vi "Set Voltage.vi"(8 "error in (no error)":errorcluster, 10 "Voltage":dbl, 11 "BenchParent in":refnum<class "BenchParent.lvclass">) -> (0 "error out":errorcluster, 3 "BenchParent out":refnum<class "BenchParent.lvclass">)   [LabVIEW 2024, in "BenchParent.lvclass"]
uses:
  BenchParent.lvclass
  BenchParent.lvclass/BenchParent.ctl
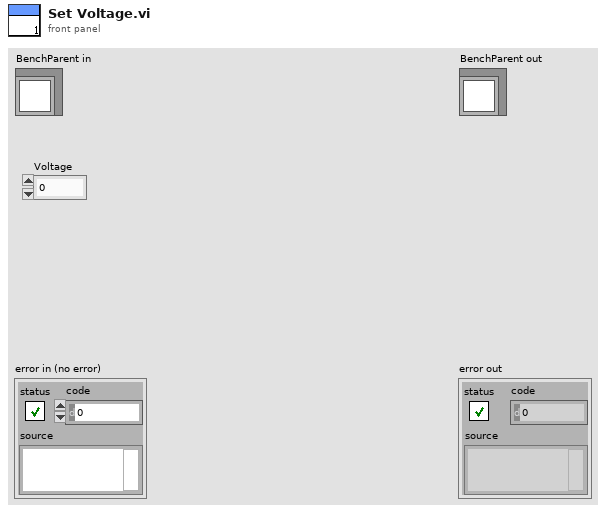
[diagram p1: front panel]
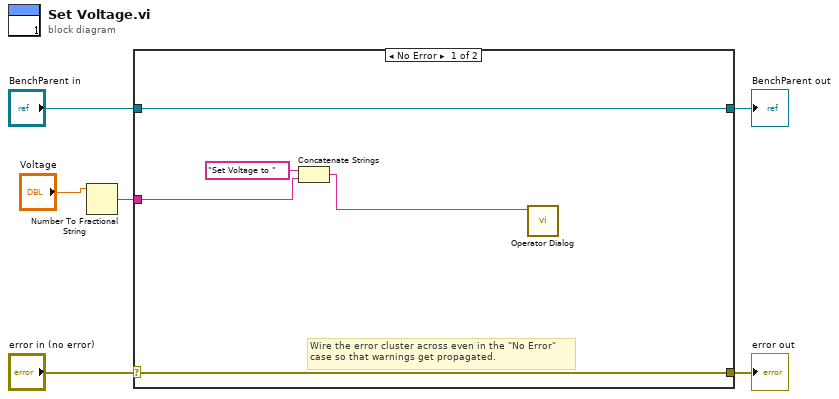
[diagram p0: block diagram]
diagram:
  n1 = Number To Fractional String(number="Voltage") -> (F-format string=w1:string)  [unwired: 3 in]
  n2 = case shown="No Error" "error in (no error)" {
    selector: "error in (no error)" -> [w10 w13]
    tunnel: [w10 w13] -> w5
    tunnel: [w11 w12] -> w3
    tunnel: "BenchParent in" -> [w11 w12]
    tunnel: w1 -> [w8 _]
    frame No Error {
      # "Wire the error cluster across even in the \"No Error\"\ncase so that warnings get propagated."
      n3 = Concatenate Strings("Set Voltage to " ("string"), w8) -> (w7:string)
      n4 = call "Operator Dialog.vi"("Message"=w7) -> ()  [unwired: 11 in]
    }
    frame Error {
    }
  }
  "error out" <- w5
  "BenchParent out" <- w3
